vi "R4SBRControl.vi"(8 "error constant":errorcluster, 11 "LabVIEW Web Service":refnum<class "Web Service.lvclass">) -> (0 "error out":errorcluster)   [LabVIEW 2016]
uses:
  <vilib>/wsapi/Web Service.lvclass
  R4Controls/R4SBR_SetParams.ctl
  <vilib>/Platform/TimedLoop/XDataNode/timing_clust.ctl
  <vilib>/Platform/TimedLoop/XDataNode/nitl_modes.ctl
  <vilib>/Platform/TimedLoop/XDataNode/wakeup.ctl
  <vilib>/Platform/TimedLoop/XDataNode/loadnilvce.vi
  <vilib>/Platform/TimedLoop/XDataNode/XDataNode.xnode
  <vilib>/Utility/Variable/NI_VariableUtilities.lvlib
  <vilib>/Platform/TimedLoop/XDataNode/XDNodeRunTimeDep.lvlib
panel:
  out "Numeric 2":i32
  out "current time":timestamp
  out "No phases":i32
  out "Numeric":i32
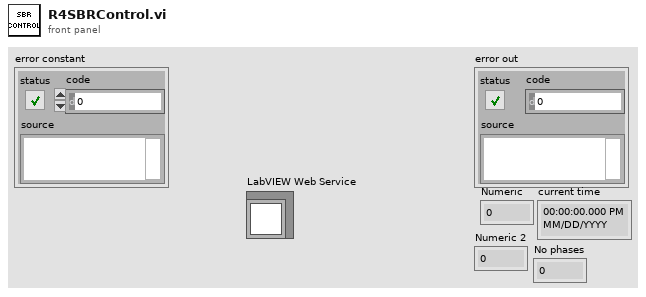
[diagram p1: front panel]
types:
  T1 = typedef "XDNodeRunTimeDep.lvlib/timing_clust.ctl" = cluster{"Expected End [f-1]":u64, "Actual End [f-1]":u64, "Finished Late? [f-1]":bool, "Expected End [i-1]":u64, "Actual End [i-1]":u64, "Finished Late? [i-1]":bool, "Expected Start [i]":u64, "Actual Start [i]":u64, "Expected Start [f]":u64, "Actual Start [f]":u64, "Source Name":string, "Structure Name":string, "Period":i64, "Deadline":i64, "Offset":i64, "Start":i64, "Priority":i32, "Timeout":i32, "Mode":T2, "Wakeup Reason":T3, "Error":errorcluster, "Source Type":string, "Secondary Source Type":string, "Global End Time":u64, "Global Start Time":u64, "Frame Duration":u64, "Iteration Duration":u64, "Assigned CPU":i32, "I/O Scan Engine Mode":u32}
  T2 = typedef "XDNodeRunTimeDep.lvlib/nitl_modes.ctl" = enum32{"No Change", "Process missed periods, maintain original phase", "Discard missed periods, maintain original phase", "Process missed periods, ignore original phase", "Discard missed periods, ignore original phase"}
  T3 = typedef "XDNodeRunTimeDep.lvlib/wakeup.ctl" = enum32{"Normal", "Aborted", "Asynchronous wakeup", "Timing source error", "Timed loop error", "Timeout"}
  T4 = cluster{"Media Pump":bool, "Water Pump":bool, "Effluent Pump":bool, "Release Valve":bool, "Gas Pump":bool}
  T5 = typedef "R4SBR_SetParams.ctl" = cluster{"Phase":string, "Time, min":dbl, "SBR_Manual (Standard)":cluster{"Media Pump":bool, "Water Pump":bool, "Gas Pump":bool, "Effluent Pump":bool, "Release Pump":bool}}[]
  T6 = cluster{"Media Pump":bool, "Water Pump":bool, "Gas Pump":bool, "Effluent Pump":bool, "Release Pump":bool}
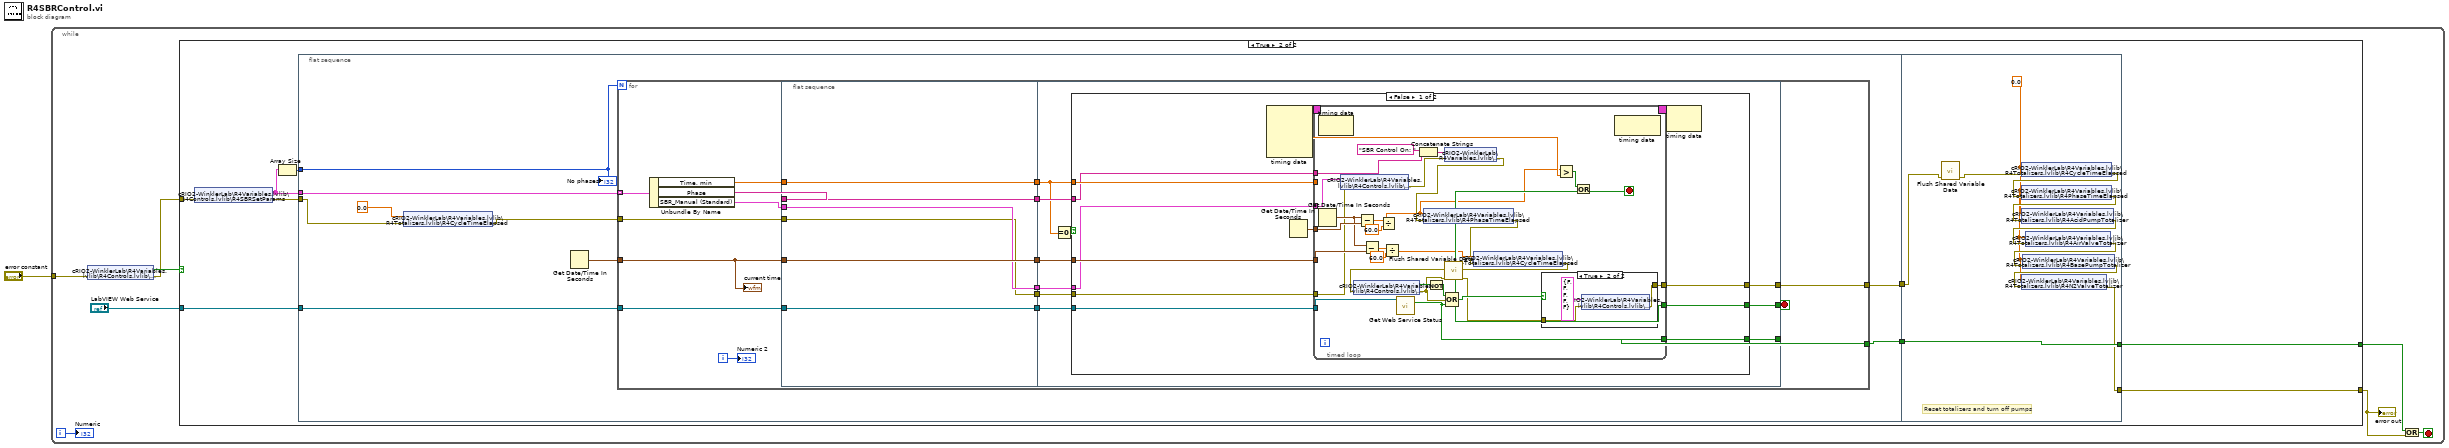
[diagram p0: block diagram]
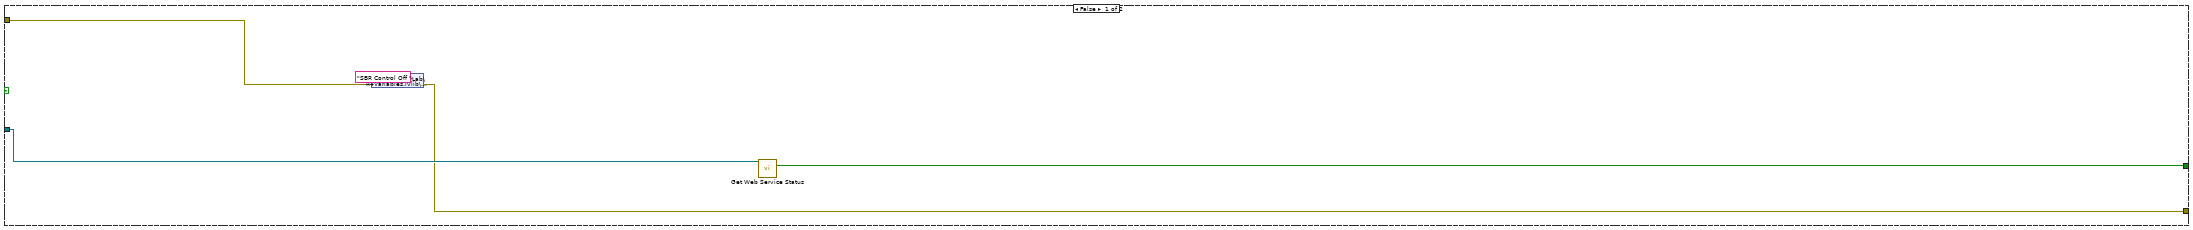
[diagram p2: hidden frame]
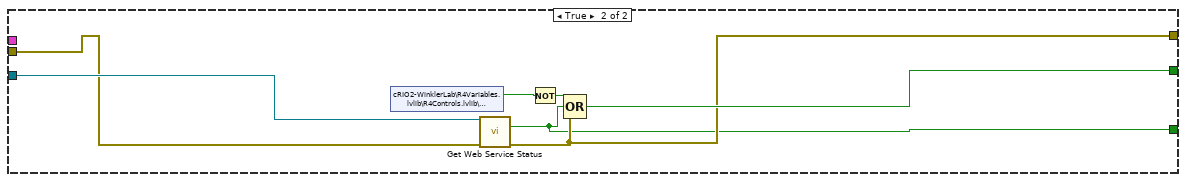
[diagram p4: hidden frame]
diagram:
  n1 = while {
    tunnel: "error constant" -> [w2]
    i -> [w6]
    stop <- w7 stop-if-true
    n2 = shared-variable "cRIO2-WinklerLab\\R4Variables.lvlib\\R4Controls.lvlib\\R4SBRSwitch"(error in=w2) -> (w4:bool, error out=w3:errorcluster)
    n3 = case shown="True" w4 {
      tunnel: "LabVIEW Web Service" -> [w14 w22]
      tunnel: w3 -> [w11 w15]
      tunnel: [w12 w18] -> w8
      tunnel: [w13 w20] -> w5
      frame False {
        n4 = shared-variable "cRIO2-WinklerLab\\R4Variables.lvlib\\R4Status"("SBR Control Off " ("string"), error in=w11) -> (error out=w12:errorcluster)
        n5 = call <vilib>:"Get Web Service Status.vi"("LabVIEW Web Service"=w14) -> ("service stopping?"=w13:bool)  [unwired: 12 in, 2 out]
      }
      frame True {
        n6 = shared-variable "cRIO2-WinklerLab\\R4Variables.lvlib\\R4Controls.lvlib\\R4SBRSetParams"(error in=w15) -> (w17:T5, error out=w16:errorcluster)
        n7 = Array Size(array=w17) -> (size(s)=w23:i32)
        n8 = flat-sequence {
          tunnel: w17 -> [w31]
          tunnel: w23 -> [w32]
          tunnel: w22 -> [w30]
          tunnel: w16 -> [w26]
          tunnel: [w28] -> w21
          tunnel: [w27] -> w19
          tunnel: w21 -> [w131]
          tunnel: [w130] -> w20
          tunnel: w19 -> [w130]
          tunnel: [w124] -> w18
          frame #0 {
            n9 = shared-variable "cRIO2-WinklerLab\\R4Variables.lvlib\\R4Totalizers.lvlib\\R4CycleTimeElapsed"(0.0 ("R1CycleTimeElapsed"), error in=w26) -> (error out=w24:errorcluster)
            n10 = Get Date/Time In Seconds() -> (seconds since 1Jan1904=w29:timestamp)
            n11 = for {
              N: w32 -> [_]
              tunnel: w31 -> [w49] mode=indexing
              tunnel: w30 -> [w48]
              tunnel: w24 -> [w42]
              tunnel: [w40] -> w28
              tunnel: w29 -> [w37]
              tunnel: [w36] -> w27
              i -> [w38]
              stop <- w39 stop-if-true
              n12 = Unbundle By Name(w49) -> ("Time, min"=w45:dbl, "Phase"=w44:string, "SBR_Manual (Standard)"=w33:T6)
              n13 = flat-sequence {
                tunnel: w45 -> [w54]
                tunnel: w33 -> [w51]
                tunnel: w48 -> [w55]
                tunnel: [w55] -> w47
                tunnel: [w54] -> w46
                tunnel: w44 -> [w53]
                tunnel: [w53] -> w43
                tunnel: w42 -> [w50]
                tunnel: w37 -> [w52]
                tunnel: [w52] -> w41
                tunnel: [w51] -> w35
                tunnel: [w50] -> w34
                tunnel: [w64] -> w39
                tunnel: w47 -> [w65]
                tunnel: w46 -> [w56]
                tunnel: w43 -> [w63]
                tunnel: w41 -> [w62]
                tunnel: [w61] -> w40
                tunnel: [w60] -> w36
                tunnel: w35 -> [w59]
                tunnel: w34 -> [w58]
                frame #0 {
                }
                frame #1 {
                  n14 = Equal To 0?(x=w56) -> (x = 0?=w57:bool)
                  n15 = case shown="False" w57 {
                    tunnel: w65 -> [w77 w120]
                    tunnel: [w76 w118] -> w64
                    tunnel: w63 -> [w66 _]
                    tunnel: w62 -> [w74 _]
                    tunnel: [w73 w117] -> w61
                    tunnel: [w72 w116] -> w60
                    tunnel: w59 -> [w67 _]
                    tunnel: w58 -> [w68 w119]
                    tunnel: w56 -> [w71 _]
                    frame False {
                      n16 = node-c288() -> (w70:T1)  [unwired: 4 in]
                      n17 = Get Date/Time In Seconds() -> (seconds since 1Jan1904=w75:timestamp)
                      n18 = timed-loop {
                        tunnel: w77 -> [w100]
                        tunnel: [w96] -> w76
                        tunnel: w75 -> [w104]
                        tunnel: w74 -> [w101]
                        tunnel: [w94] -> w73
                        tunnel: [w97] -> w72
                        tunnel: w68 -> [w82]
                        tunnel: w71 -> [w93]
                        timing: w70 -> [_]
                        timing-out: [_] -> w69
                        tunnel: w67 -> [w81]
                        tunnel: w66 -> [w89]
                        stop <- w92 stop-if-true
                        n19 = node-c288() -> ()  [unwired: 1 in, 1 out]
                        n20 = Get Date/Time In Seconds() -> (seconds since 1Jan1904=w102:timestamp)
                        n21 = shared-variable "cRIO2-WinklerLab\\R4Variables.lvlib\\R4Controls.lvlib\\R4SBRManual"(w81, error in=w82) -> (error out=w83:errorcluster)
                        n22 = Subtract(x=w102, y=w104) -> (x-y=w105:dbl)
                        n23 = Subtract(x=w102, y=w101) -> (x-y=w99:dbl)
                        n24 = Divide(x=w105, y=60.0) -> (x/y=w86:dbl)
                        n25 = Divide(x=w99, y=60.0) -> (x/y=w88:dbl)
                        n26 = call <vilib>:"Get Web Service Status.vi"("LabVIEW Web Service"=w100) -> ("service stopping?"=w97:bool)  [unwired: 12 in, 2 out]
                        n27 = Concatenate Strings("SBR Control On: " ("string"), w89) -> (w84:string)
                        n28 = shared-variable "cRIO2-WinklerLab\\R4Variables.lvlib\\R4Status"(w84, error in=w83) -> (error out=w85:errorcluster)
                        n29 = shared-variable "cRIO2-WinklerLab\\R4Variables.lvlib\\R4Totalizers.lvlib\\R4PhaseTimeElapsed"(w86, error in=w85) -> (error out=w87:errorcluster)
                        n30 = shared-variable "cRIO2-WinklerLab\\R4Variables.lvlib\\R4Totalizers.lvlib\\R4CycleTimeElapsed"(w88, error in=w87) -> (error out=w80:errorcluster)
                        n31 = shared-variable "cRIO2-WinklerLab\\R4Variables.lvlib\\R4Controls.lvlib\\R4SBRSwitch"(error in=w80) -> (w79:bool, error out=w78:errorcluster)
                        n32 = Not(x=w79) -> (.not. x?=w106:bool)
                        n33 = call <vilib>:"Flush Shared Variable Data.vi"("error in (no error)"=w78) -> ("error out"=w95:errorcluster)  [unwired: 10 in]
                        n34 = Compound Arithmetic op=OR(w106, w78, w97) -> (w96:bool)
                        n35 = case shown="True" w96 {
                          tunnel: w95 -> [w109 w111]
                          tunnel: [w109 w112] -> w94
                          frame False {
                          }
                          frame True {
                            n36 = shared-variable "cRIO2-WinklerLab\\R4Variables.lvlib\\R4Controls.lvlib\\R4SBRManual"(T4 {"Media Pump"=FALSE, "Water Pump"=FALSE, "Effluent Pump"=FALSE, "Release Valve"=FALSE, "Gas Pump"=FALSE} ("R1SBRManual"), error in=w111) -> (error out=w112:errorcluster)
                          }
                        }
                        n37 = Greater?(x=w86, y=w93) -> (0:w91:bool)
                        n38 = Or(x=w91, y=w96) -> (x .or. y?=w92:bool)
                        n39 = node-c288() -> ()  [unwired: 1 in, 1 out]
                      }
                      n40 = node-c288(w69) -> ()  [unwired: 1 out]
                    }
                    frame True {
                      n41 = shared-variable "cRIO2-WinklerLab\\R4Variables.lvlib\\R4Controls.lvlib\\R4SBRSwitch"() -> (w115:bool)  [unwired: 1 in, 1 out]
                      n42 = call <vilib>:"Get Web Service Status.vi"("LabVIEW Web Service"=w120, "error in (no error)"=w119) -> ("service stopping?"=w116:bool, "error out"=w117:errorcluster)  [unwired: 11 in, 1 out]
                      n43 = Not(x=w115) -> (.not. x?=w121:bool)
                      n44 = Compound Arithmetic op=OR(w121, w116, w117) -> (w118:bool)
                    }
                  }
                }
              }
              "Numeric 2" <- w38
              "current time" <- w37
            }
            "No phases" <- w32
          }
          frame #1 {
            w122 = 0.0 ("R1CycleTimeElapsed")
            # "Reset totalizers and turn off pumps"
            n45 = call <vilib>:"Flush Shared Variable Data.vi"("error in (no error)"=w131) -> ("error out"=w123:errorcluster)  [unwired: 10 in]
            n46 = shared-variable "cRIO2-WinklerLab\\R4Variables.lvlib\\R4Totalizers.lvlib\\R4CycleTimeElapsed"(w122, error in=w123) -> (error out=w129:errorcluster)
            n47 = shared-variable "cRIO2-WinklerLab\\R4Variables.lvlib\\R4Totalizers.lvlib\\R4PhaseTimeElapsed"(w122, error in=w129) -> (error out=w128:errorcluster)
            n48 = shared-variable "cRIO2-WinklerLab\\R4Variables.lvlib\\R4Totalizers.lvlib\\R4AcidPumpTotalizer"(w122, error in=w128) -> (error out=w127:errorcluster)
            n49 = shared-variable "cRIO2-WinklerLab\\R4Variables.lvlib\\R4Totalizers.lvlib\\R4AirValveTotalizer"(w122, error in=w127) -> (error out=w126:errorcluster)
            n50 = shared-variable "cRIO2-WinklerLab\\R4Variables.lvlib\\R4Totalizers.lvlib\\R4BasePumpTotalizer"(w122, error in=w126) -> (error out=w125:errorcluster)
            n51 = shared-variable "cRIO2-WinklerLab\\R4Variables.lvlib\\R4Totalizers.lvlib\\R4N2ValveTotalizer"(w122, error in=w125) -> (error out=w124:errorcluster)
          }
        }
      }
    }
    "error out" <- w8
    n52 = Or(x=w5, y=w8) -> (x .or. y?=w7:bool)
    "Numeric" <- w6
  }
